vi "Find Elements by Name.vi"(1 "name":string, 2 "XML Elements":T1[](array[typedef])) -> (0 "XML Elements":T1[](array[typedef]))   [LabVIEW 2011]
uses:
  Type Defs/XML Element Table - Cluster.ctl
  Type Defs/Node Info - Cluster.ctl
  <userlib>/_OpenG.lib/array/array.llb/Search 1D Array (String)__ogtk.vi
  <userlib>/_OpenG.lib/array/array.llb/Index 1D Array Elements (Variant)__ogtk.vi
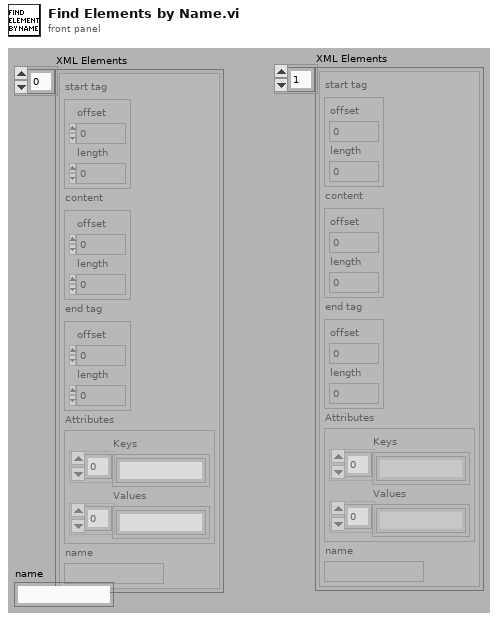
[diagram p1: front panel]
types:
  T1 = typedef "XML Element Table - Cluster.ctl" = cluster{"start tag":T2, "content":T2, "end tag":T2, "Attributes":cluster{"Keys":string[], "Values":string[]}, "name":string}
  T2 = typedef "Node Info - Cluster.ctl" = cluster{"offset":i32, "length":i32}
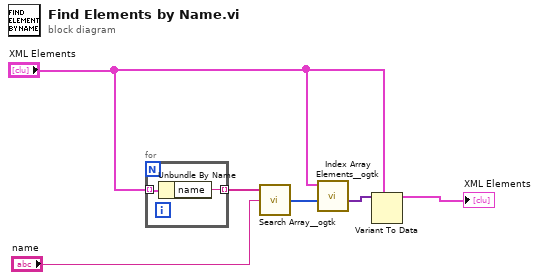
[diagram p0: block diagram]
diagram:
  n1 = for {
    tunnel: "XML Elements" -> [w8] mode=indexing
    tunnel: [w7] -> w6 mode=indexing
    n2 = Unbundle By Name(w8) -> ("name"=w7:string)
  }
  n3 = call-poly <userlib>:"Search Array__ogtk.vi"("Array"=w6, "Element Data"="name") -> ("Indices of Elements"=w1:i32[])  [unwired: 7 in]
  n4 = call-poly <userlib>:"Index Array Elements__ogtk.vi"("indices"=w1, "array"="XML Elements") -> ("elements"=w2:variant[])  [unwired: 9 in]
  n5 = Variant To Data(type="XML Elements", Variant=w2) -> (data=→"XML Elements":T1[])  [unwired: 1 in, 1 out]
